vi "Obtain Session.vi"(0 "Session  Name ()":string, 7 "DUMMY data":bool, 11 "error in (no error)":errorcluster) -> (4 "Session Handle":T1, 15 "error out":errorcluster)   [LabVIEW 2016, in "Template Session.lvclass"]
doc: "This function initializes the measurement\n\nPass the function a name to obtain an active measurement handle"
uses:
  Template Session.lvclass
  Session - Root.lvclass
  F:/Dropbox/sw_repo/For Builds/Reusable/Session APIs/_Session Fwk/Session - Root.lvclass
  Typedefs/Session Handle.ctl
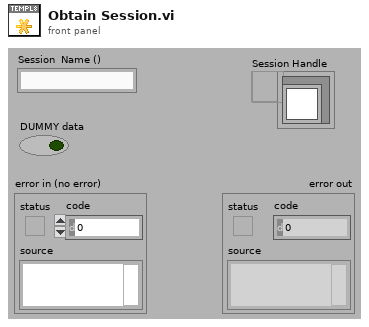
[diagram p1: front panel]
types:
  T1 = typedef "Template Session.lvclass/Session Handle.ctl" = refnum<data-value>
  T2 = typedef "Session - Root.lvclass/Session Handle.ctl" = refnum<data-value>
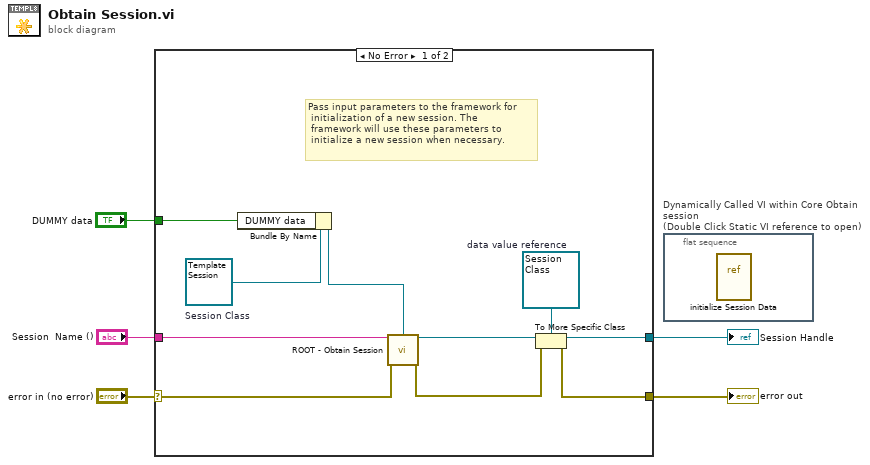
[diagram p0: block diagram]
diagram:
  n1 = case shown="No Error" "error in (no error)" {
    selector: "error in (no error)" -> [w14 w16]
    tunnel: [w11 w16] -> w4
    tunnel: [w13 _] -> w1
    tunnel: "Session  Name ()" -> [w15 _]
    tunnel: "DUMMY data" -> [w8 _]
    frame No Error {
      w6 = refnum<data-value> refnum  # data value reference
      w7 = refnum<class "Template Session.lvclass"> refnum  # Session Class
      # "Pass input parameters to the framework for\n initialization of a new session. The\n framework will use these parameters to\n initialize a new session when necessary."
      n2 = Bundle By Name(cluster=w7, "DUMMY data"=w8) -> (w9:refnum<class "Template Session.lvclass">)
      n3 = call "ROOT - Obtain Session.vi"("Session Name ()"=w15, "OBJ - Session"=w9, "error in (no error)"=w14) -> ("Session Handle"=w10:T2, "error out"=w12:errorcluster)  [unwired: 10 in, 1 out]
      n4 = To More Specific Class(target class=w6, reference=w10, error in=w12) -> (specific class reference=w13:refnum<data-value>, error out=w11:errorcluster)
    }
    frame Error {
    }
  }
  "error out" <- w4
  "Session Handle" <- w1
  n5 = flat-sequence "Dynamically Called VI within Core Obtain session\n(Double Click Static VI reference to open)" {
    frame #0 {
      n6 = vi-ref "initialize Session Data.vi"() -> ()  [unwired: 1 out]
    }
  }
